vi "Generate Library Icon.vi"(8 "error in (no error)":errorcluster, 10 "Library Path":path, 11 "App Reference":refnum<vi>) -> (0 "error out":errorcluster, 3 "App Reference Out":refnum<vi>)   [LabVIEW 2020, in "Project Provider.lvlib"]
uses:
  <vilib>/LabVIEW Icon API/lv_icon/classes/Icon/Icon.lvclass
  <vilib>/LabVIEW Icon API/API_Rectangle Dimension.ctl
  <vilib>/LabVIEW Icon API/API_Text.ctl
  <vilib>/LabVIEW Icon API/API_Rectangle Colors.ctl
  Project Provider.lvlib
  <vilib>/LabVIEW Icon API/LabVIEW Icon API.lvlib
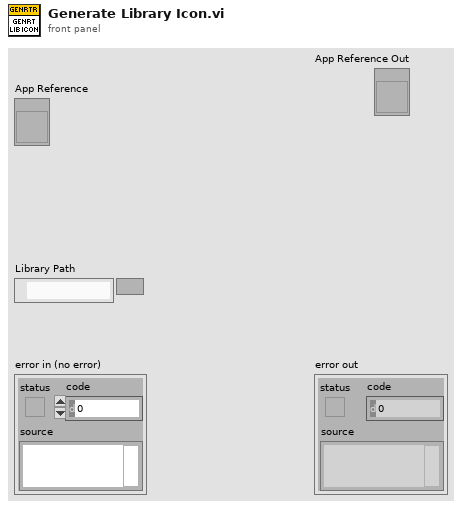
[diagram p1: front panel]
types:
  T1 = typedef "LabVIEW Icon API.lvlib/API_Rectangle Colors.ctl" = cluster{"Border":u32, "Background":u32}
  T2 = typedef "LabVIEW Icon API.lvlib/API_Text.ctl" = cluster{"Line 1 text":string, "Line 2 text":string, "Line 3 text":string, "Line 4 text":string}
  T3 = typedef "LabVIEW Icon API.lvlib/API_Rectangle Dimension.ctl" = cluster{"Width":i16, "Height":i16}
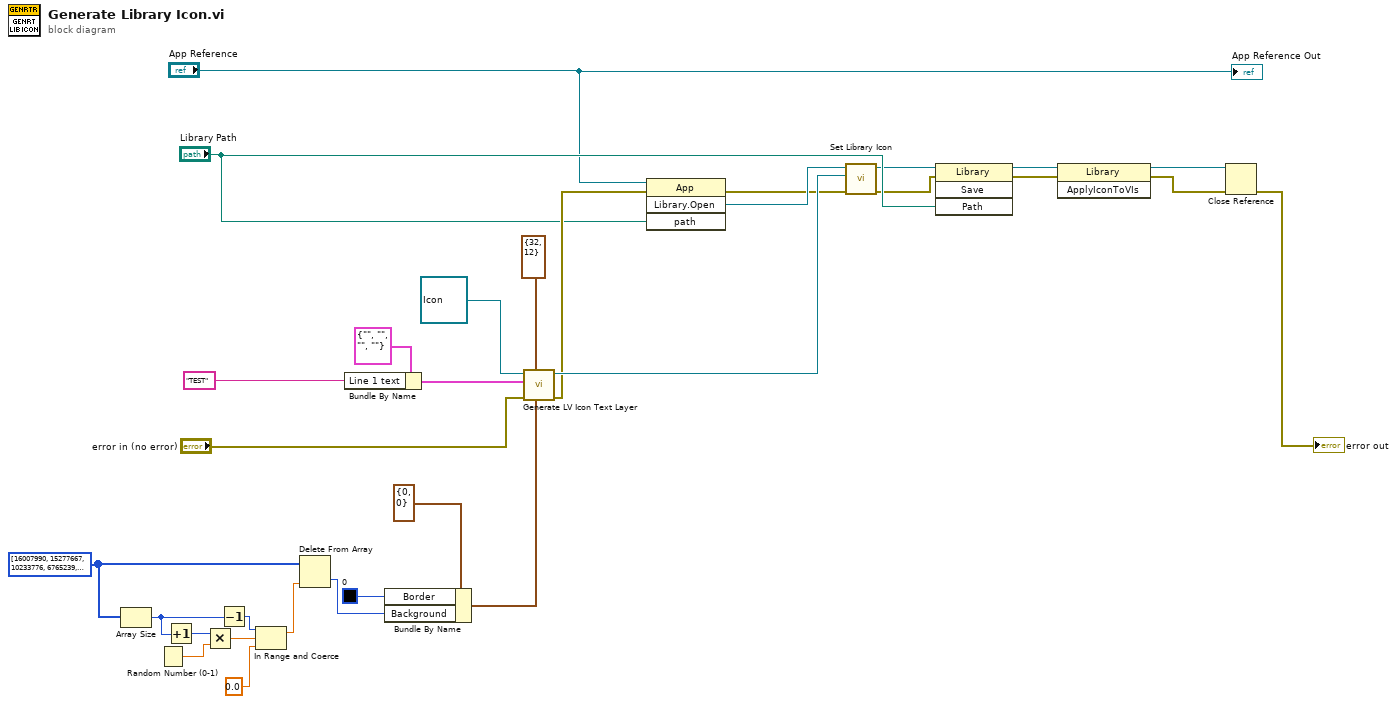
[diagram p0: block diagram]
diagram:
  w12 = u32[] [16007990, 15277667, 10233776, 6765239, 4149685, 2201331, 240116, 48340, 38536, 5025616, 9159498, 13491257, 16771899, 16761095, 16750592, 16733986, 7951688, 10395294, 6323595] ("Array")
  n1 = Array Size(array=w12) -> (size(s)=w6:i32)
  n2 = Random Number (0-1)() -> (number: 0 to 1=w5:dbl)
  n3 = Increment(x=w6) -> (x+1=w7:i32)
  n4 = Multiply(x=w7, y=w5) -> (x*y=w10:dbl)
  n5 = Decrement(x=w6) -> (x-1=w9:i32)
  n6 = In Range and Coerce(upper limit=w9, x=w10, lower limit=0.0) -> (coerced(x)=w4:dbl)  [unwired: 1 out]
  n7 = Delete From Array(array=w12, index=w4) -> (deleted portion=w11:u32)  [unwired: 1 in, 1 out]
  n8 = Bundle By Name(cluster=T2 {"Line 1 text"="", "Line 2 text"="", "Line 3 text"="", "Line 4 text"=""} ("Text"), "Line 1 text"="TEST" ("Overlay Text")) -> (w27:T2)
  n9 = Bundle By Name(cluster=T1 {"Border"=0, "Background"=0} ("Library Color"), "Border"=u32 0 ("Background"), "Background"=w11) -> (w13:T1)
  n10 = call <vilib>:"Generate LV Icon Text Layer.vi"("Rectangle colors (black, white)"=w13, "Rectangle dimension (32,32)"=T3 {"Width"=32, "Height"=12}, "error in (no error)"="error in (no error)", "Text"=w27, "Icon in"=refnum<class "Icon.lvclass"> refnum ("Icon.lvclass in")) -> ("error out"=w23:errorcluster, "Icon out"=w28:refnum<class "Icon.lvclass">)  [unwired: 5 in]
  n11 = invoke class="App" method="Library.Open"(reference="App Reference", error in=w23, "path"="Library Path") -> (error out=w19:errorcluster, "Open Library"=w21:refnum<vi>)  [unwired: 1 in, 2 out]
  n12 = call <vilib>:"Set Library Icon.vi"("error in (no error)"=w19, "Icon"=w28, "Library Refnum in"=w21) -> ("error out"=w18:errorcluster, "Library Refnum out"=w20:refnum<vi>)  [unwired: 7 in]
  n13 = invoke class="Library" method="Save"(reference=w20, error in=w18, "Path"="Library Path") -> (reference out=w2:refnum<vi>, error out=w17:errorcluster)  [unwired: 1 in, 2 out]
  n14 = invoke class="Library" method="ApplyIconToVIs"(reference=w2, error in=w17) -> (reference out=w1:refnum<vi>, error out=w3:errorcluster)  [unwired: 1 in, 1 out]
  n15 = Close Reference(reference=w1, error in (no error)=w3) -> (error out=→"error out":errorcluster)
  "App Reference Out" <- "App Reference"
